vi "aleatoriop.vi"() -> ()   [LabVIEW 2020]
panel:
  in  "Tab Control":enum32{"numeros aleatorios k"}(tab)
  in  "Delay ms":dbl(slide) scale=10.0..4000.0
  in  "STOP":bool
  out "k Base 11":string
  out "k Base 4":i32
  out "k Decimal":dbl
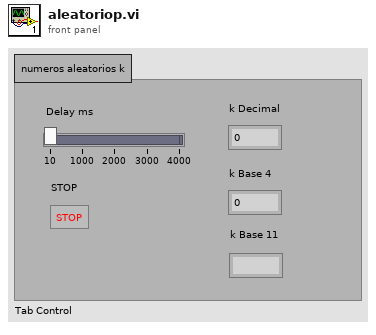
[diagram p1: front panel]
types:
  T1 = enum16{"open", "replace", "create", "open or create", "replace or create", "replace or create with confirmation"}
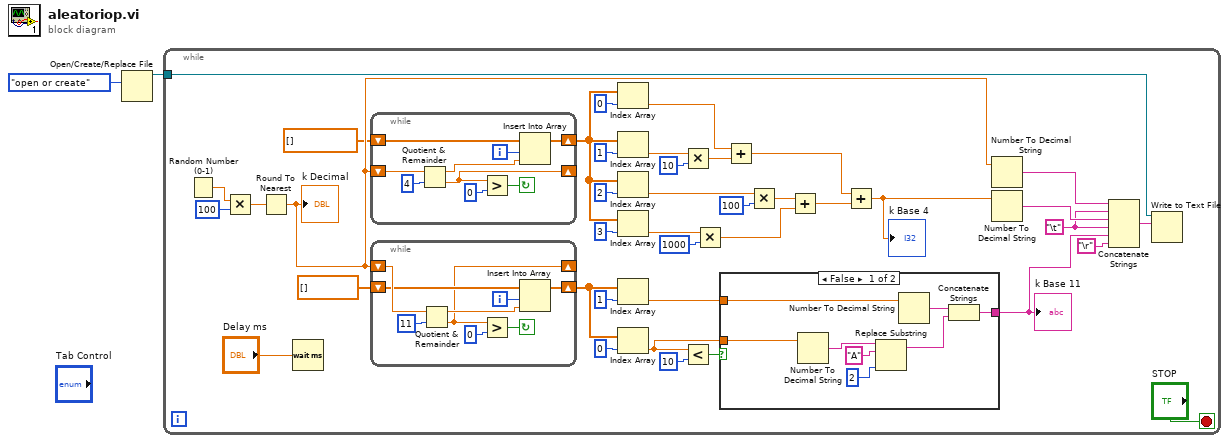
[diagram p0: block diagram]
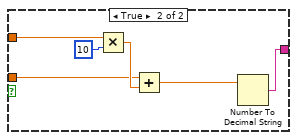
[diagram p2: hidden frame]
diagram:
  n1 = Open/Create/Replace File(operation (0:open)=T1."open or create") -> (refnum out=w1:refnum<file>)  [unwired: 5 in, 2 out]
  n2 = while {
    tunnel: w1 -> [w18]
    stop <- "STOP" stop-if-true
    w11 = "\t"
    n3 = Random Number (0-1)() -> (number: 0 to 1=w16:dbl)
    n4 = Multiply(x=w16, y=100) -> (x*y=w14:dbl)
    n5 = Round To Nearest(number=w14) -> (nearest integer value=w13:dbl)
    "k Decimal" <- w13
    n6 = Wait (ms)(milliseconds to wait="Delay ms") -> ()  [unwired: 1 out]
    n7 = while {
      shift-right: [w61] -> w20
      shift-left: dbl[] [] -> [w60]
      shift-right: [w58] -> _
      shift-left: w13 -> [w64]
      i -> [w59]
      stop <- w63 continue-if-true
      n8 = Quotient & Remainder(x=w64, y=4) -> (x-y*floor(x/y)=w57:dbl, floor(x/y)=w58:dbl)
      n9 = Greater?(x=w58, y=0) -> (0:w63:bool)
      n10 = Insert Into Array(array=w60, index=w59, new element=w57) -> (w61:dbl[])
    }
    n11 = while {
      shift-right: [w72] -> w40
      shift-left: dbl[] [] -> [w71]
      shift-right: [w67] -> _
      shift-left: w13 -> [w74]
      i -> [w73]
      stop <- w66 continue-if-true
      n12 = Quotient & Remainder(x=w74, y=11) -> (x-y*floor(x/y)=w70:dbl, floor(x/y)=w67:dbl)
      n13 = Greater?(x=w67, y=0) -> (0:w66:bool)
      n14 = Insert Into Array(array=w71, index=w73, new element=w70) -> (w72:dbl[])
    }
    n15 = Index Array(array=w20, index=0) -> (element=w38:dbl)
    n16 = Index Array(array=w20, index=1) -> (element=w36:dbl)
    n17 = Index Array(array=w20, index=2) -> (element=w31:dbl)
    n18 = Index Array(array=w20, index=3) -> (element=w30:dbl)
    n19 = Index Array(array=w40, index=1) -> (element=w5:dbl)
    n20 = Index Array(array=w40, index=0) -> (element=w6:dbl)
    n21 = Multiply(x=w36, y=10) -> (x*y=w39:dbl)
    n22 = Less?(x=w6, y=10) -> (x < y?=w8:bool)
    n23 = Multiply(x=w30, y=1000) -> (x*y=w27:dbl)
    n24 = case shown="False" w8 {
      tunnel: w6 -> [w47 w53]
      tunnel: w5 -> [w46 w52]
      tunnel: [w45 w51] -> w4
      frame False {
        n25 = Number To Decimal String(number=w47) -> (decimal integer string=w48:string)  [unwired: 1 in]
        n26 = Replace Substring(2:2 ("length (len. of substring)"), 4:"A", 5:w48) -> (1:w44:string)  [unwired: 1 in, 1 out]
        n27 = Number To Decimal String(number=w46) -> (decimal integer string=w43:string)  [unwired: 1 in]
        n28 = Concatenate Strings(w43, w44) -> (w45:string)
      }
      frame True {
        n29 = Multiply(x=w52, y=10) -> (x*y=w55:dbl)
        n30 = Add(x=w53, y=w55) -> (x+y=w54:dbl)
        n31 = Number To Decimal String(number=w54) -> (decimal integer string=w51:string)  [unwired: 1 in]
      }
    }
    "k Base 11" <- w4
    n32 = Add(x=w38, y=w39) -> (x+y=w24:dbl)
    n33 = Multiply(x=w31, y=100) -> (x*y=w26:dbl)
    n34 = Add(x=w26, y=w27) -> (x+y=w25:dbl)
    n35 = Add(x=w24, y=w25) -> (x+y=w23:dbl)
    "k Base 4" <- w23
    n36 = Number To Decimal String(number=w13) -> (decimal integer string=w22:string)  [unwired: 1 in]
    n37 = Number To Decimal String(number=w23) -> (decimal integer string=w21:string)  [unwired: 1 in]
    n38 = Concatenate Strings(w22, w11, w21, w11, w4, "\r") -> (w19:string)
    n39 = Write to Text File(file (use dialog)=w18, text=w19) -> ()  [unwired: 2 in, 3 out]
  }
